vi "MCSTopLevel.vi"(0 "MCSSelectTrigger":T1, 2 "delay(ticks)":u32, 5 "nOfBins":u32) -> ()   [LabVIEW 2014]
uses:
  Controls/MCSselectTrigger.ctl
  <vilib>/Platform/TimedLoop/XDataNode/timing_clust.ctl
  <vilib>/Platform/TimedLoop/XDataNode/nitl_modes.ctl
  <vilib>/Platform/TimedLoop/XDataNode/wakeup.ctl
  <vilib>/rvi/Emulation/niFpgaGetClockAttributes.vi
  <vilib>/rvi/Emulation/niFpgaSctlEmulationGetInTimedLoop.vi
  <vilib>/rvi/Emulation/niFpgaEmulationReportErrorSimple.vi
  <vilib>/rvi/Emulation/niFpgaCriticalErrorInLSC.vi
  <vilib>/rvi/Emulation/niFpgaEmulationIsFPGAContextNoSignature.vi
  <vilib>/rvi/DataTransferAndStorage/Container/Common/niFpgaContainerGetUniqueNameForEmu.vi
  <vilib>/rvi/eio/common/nirviEmuReportErrorAndStop.vi
  <vilib>/rvi/Emulation/niFpgaProcessEmulError.vi
  <vilib>/Platform/TimedLoop/XDataNode/XDataNode.xnode
  <vilib>/rvi/DataTransferAndStorage/Container/XNode/niFpgaContainer.xnode
  <vilib>/rvi/DataTransferAndStorage/Handshake/Emulation/niFpgaHandshakeEmulation.vi
  <vilib>/Platform/TimedLoop/XDataNode/XDNodeRunTimeDep.lvlib
panel:
  in  "nOfBunches":i32
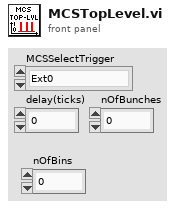
[diagram p1: front panel]
types:
  T1 = typedef "MCSselectTrigger.ctl" = enum8{"Ext0", "Ext1", "Ext2", "Ext3", "Ext4", "Ext5", "Ext6", "Ext7", "Int0", "Int1", "Int2", "Int3", "Int4", "Int5", "Int6", "Int7"}
  T2 = typedef "XDNodeRunTimeDep.lvlib/timing_clust.ctl" = cluster{"Expected End [f-1]":u64, "Actual End [f-1]":u64, "Finished Late? [f-1]":bool, "Expected End [i-1]":u64, "Actual End [i-1]":u64, "Finished Late? [i-1]":bool, "Expected Start [i]":u64, "Actual Start [i]":u64, "Expected Start [f]":u64, "Actual Start [f]":u64, "Source Name":string, "Structure Name":string, "Period":i64, "Deadline":i64, "Offset":i64, "Start":i64, "Priority":i32, "Timeout":i32, "Mode":T3, "Wakeup Reason":T4, "Error":errorcluster, "Source Type":string, "Secondary Source Type":string, "Global End Time":u64, "Global Start Time":u64, "Frame Duration":u64, "Iteration Duration":u64, "Assigned CPU":i32, "I/O Scan Engine Mode":u32}
  T3 = typedef "XDNodeRunTimeDep.lvlib/nitl_modes.ctl" = enum32{"No Change", "Process missed periods, maintain original phase", "Discard missed periods, maintain original phase", "Process missed periods, ignore original phase", "Discard missed periods, ignore original phase"}
  T4 = typedef "XDNodeRunTimeDep.lvlib/wakeup.ctl" = enum32{"Normal", "Aborted", "Asynchronous wakeup", "Timing source error", "Timed loop error", "Timeout"}
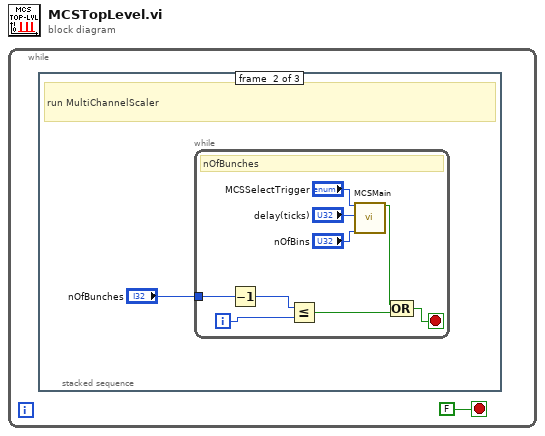
[diagram p0: block diagram]
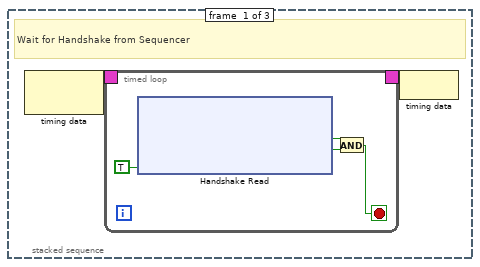
[diagram p2: hidden frame]
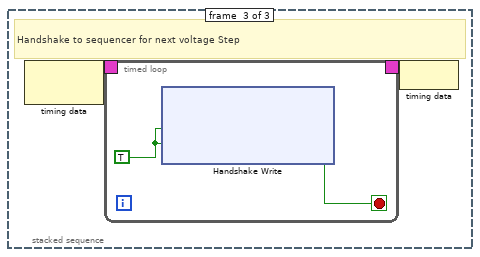
[diagram p3: hidden frame]
diagram:
  n1 = while {
    stop <- FALSE stop-if-true
    n2 = stacked-sequence {
      frame #0 {
        # "Wait for Handshake from Sequencer"
        n3 = node-c288() -> (w3:T2)  [unwired: 1 in]
        n4 = timed-loop {
          timing: w3 -> [_]
          timing-out: [_] -> w2
          stop <- w4 stop-if-true
          n5 = xnode ("Handshake Read")("Ready for Output"=TRUE) -> ("Data"=w6:bool, "Output Valid"=w5:bool)  [unwired: 1 in, 1 out]
          n6 = And(x=w6, y=w5) -> (x .and. y?=w4:bool)
        }
        n7 = node-c288(w2) -> ()
      }
      frame #1 {
        # "run MultiChannelScaler"
        n8 = while {
          tunnel: "nOfBunches" -> [w16]
          i -> [w18]
          stop <- w15 stop-if-true
          # "nOfBunches"
          n9 = Decrement(x=w16) -> (x-1=w17:i32)
          n10 = Less Or Equal?(x=w17, y=w18) -> (x <= y?=w13:bool)
          n11 = call "MCSMain.vi"("MCSSelectTrigger"="MCSSelectTrigger", "delay(ticks)"="delay(ticks)", "nOfBins"="nOfBins") -> ("abortOrTimeOut"=w14:bool)  [unwired: 16 in]
          n12 = Compound Arithmetic op=OR(w14, w13) -> (w15:bool)
        }
      }
      frame #2 {
        # "Handshake to sequencer for next voltage Step"
        n13 = node-c288() -> (w23:T2)  [unwired: 1 in]
        n14 = timed-loop {
          timing: w23 -> [_]
          timing-out: [_] -> w22
          stop <- w25 stop-if-true
          w24 = TRUE ("Ready for Output")
          n15 = xnode ("Handshake Write")("Data"=w24, "Input Valid"=w24) -> ("Ready for Input"=w25:bool)  [unwired: 1 in, 1 out]
        }
        n16 = node-c288(w22) -> ()
      }
    }
  }
